vi "Tabulate 1D Array.vi"(11 "1D Array":string[](array[string])) -> (3 "Tabulated Array":string[](array[string]))   [LabVIEW 2010]
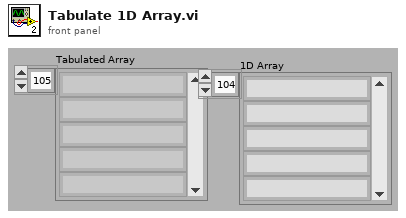
[diagram p1: front panel]
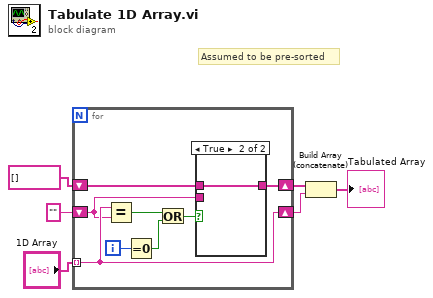
[diagram p0: block diagram]
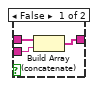
[diagram p2: hidden frame]
diagram:
  # "Assumed to be pre-sorted"
  n1 = for {
    tunnel: "1D Array" -> [w8] mode=indexing
    shift-right: [w8] -> w6
    shift-left: "" ("String") -> [w7]
    shift-right: [w14] -> w5
    shift-left: string[] [] -> [w13]
    i -> [w12]
    n2 = Equal?(x=w8, y=w7) -> (x = y?=w10:bool)
    n3 = Equal To 0?(x=w12) -> (x = 0?=w11:bool)
    n4 = Or(x=w10, y=w11) -> (x .or. y?=w9:bool)
    n5 = case shown="True" w9 {
      tunnel: [w17 w18] -> w14
      tunnel: w13 -> [w16 w18]
      tunnel: w7 -> [w15 _]
      frame False {
        n6 = Build Array (concatenate)(w16, w15) -> (w17:string[])
      }
      frame True {
      }
    }
  }
  n7 = Build Array (concatenate)(w5, w6) -> (→"Tabulated Array":string[])
